vi "Localize CSM VIs.vi"(5 "API Dir":path[](array[path]), 6 "options":cluster{"Force?(F)":bool, "Show FP":bool}={"Force?(F)"=FALSE, "Show FP"=TRUE}, 7 "doc dir":path[](array[path]), 8 "error in (no error)":errorcluster, 10 "Language Ring":string(combo)="English(en-us)") -> (0 "error out":errorcluster)   [LabVIEW 2017, in "csmdoc.lvlib"]
uses:
  csmdoc.lvlib
  BEditor-Localization.vi
  _Typedef/DocElement.ctl
  _Shared/CSM Shared.lvlib
  _tool/_batchEditorDialog/batchEditorDialog.lvlib
  Communicable State Machine.lvlib
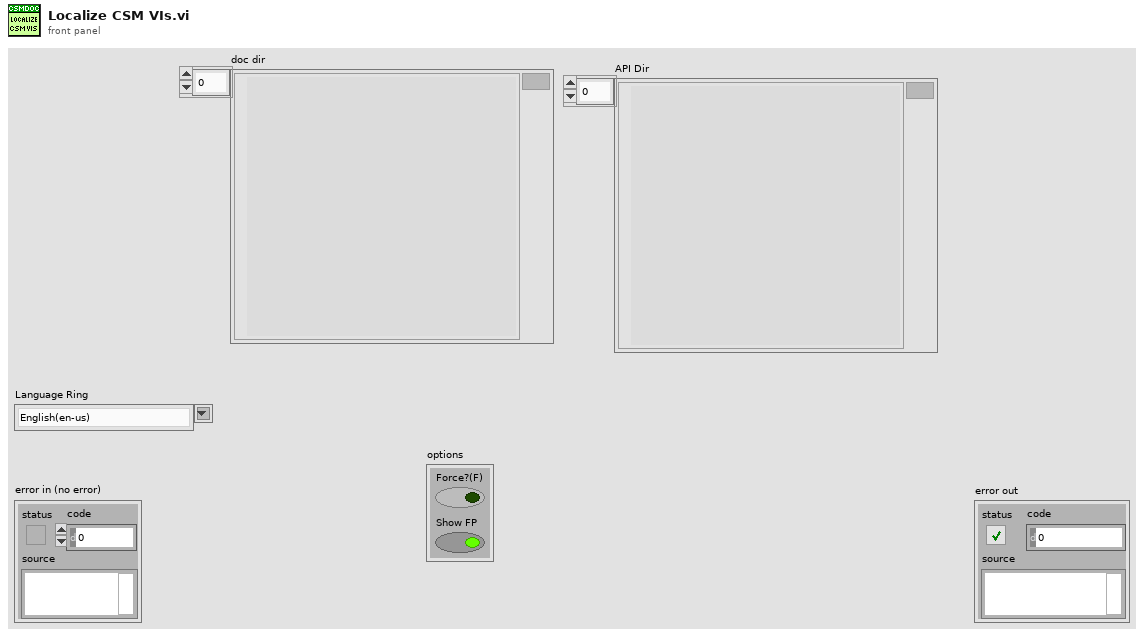
[diagram p1: front panel]
types:
  T1 = typedef "csmdoc.lvlib/DocNote.ctl" = cluster{"ID":string, "Content":string, "Type":string}
  T2 = typedef "csmdoc.lvlib/DocElement.ctl" = cluster{"ID":string, "Content":string[], "SubIDs":string[], "Path":string[]}
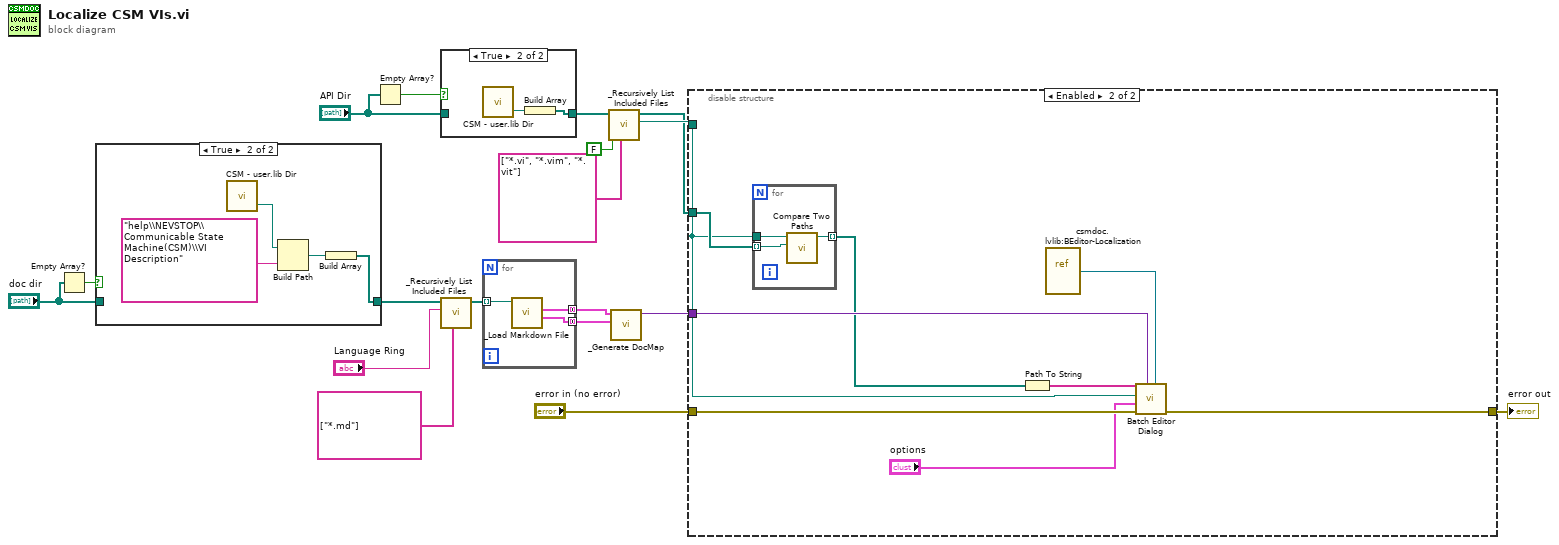
[diagram p0: block diagram]
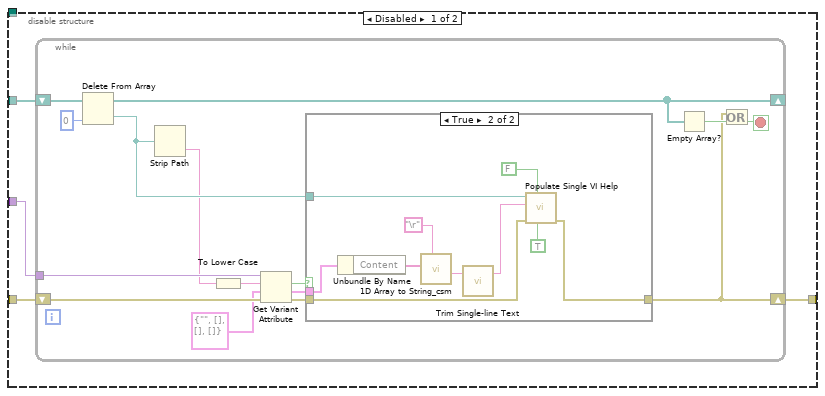
[diagram p2: hidden frame]
diagram:
  n1 = Empty Array?(array="doc dir") -> (empty?=w12:bool)
  n2 = case shown="True" w12 {
    tunnel: [w19 w20] -> w18
    tunnel: "doc dir" -> [w19 _]
    frame False {
    }
    frame True {
      n3 = call "CSM - user.lib Dir.vi"() -> ("<LabVIEW>"=w21:path)  [unwired: 2 in, 1 out]
      n4 = Build Path(base path=w21, name or relative path="help\\NEVSTOP\\Communicable State Machine(CSM)\\VI Description") -> (appended path=w22:path)
      n5 = Build Array(w22) -> (w20:path[])
    }
  }
  n6 = Empty Array?(array="API Dir") -> (empty?=w10:bool)
  n7 = case shown="True" w10 {
    tunnel: "API Dir" -> [w24 _]
    tunnel: [w24 w25] -> w3
    frame False {
    }
    frame True {
      n8 = call "CSM - user.lib Dir.vi"() -> ("<LabVIEW>"=w26:path)  [unwired: 2 in, 1 out]
      n9 = Build Array(w26) -> (w25:path[])
    }
  }
  n10 = call "_Recursively List Included Files.vi"("pattern"=string[] ["*.md"], "Language Ring"="Language Ring", "dir"=w18) -> ("Array"=w15:path[])  [unwired: 7 in, 1 out]
  n11 = for {
    tunnel: w15 -> [w29] mode=indexing
    tunnel: [w28] -> w17 mode=concatenating
    tunnel: [w27] -> w16 mode=concatenating
    n12 = call "_Load Markdown File.vi"("Path"=w29) -> ("Array 2"=w27:T1[], "Array"=w28:T2[])  [unwired: 8 in, 1 out]
  }
  n13 = call "_Recursively List Included Files.vi"("pattern"=string[] ["*.vi", "*.vim", "*.vit"], "apply _ filter?(T)"=FALSE, "dir"=w3) -> ("Common Path"=w6:path, "Array"=w4:path[])  [unwired: 7 in]
  n14 = call "_Generate DocMap.vi"("Array 2"=w16, "Array"=w17) -> ("Variant"=w13:variant)  [unwired: 9 in]
  n15 = disable-structure shown="Enabled" {
    disable-tunnel: [w33 w67] -> w14
    disable-tunnel: "error in (no error)" -> [w32 w68]
    disable-tunnel: w13 -> [w31 w66]
    disable-tunnel: w4 -> [w30 w62]
    disable-tunnel: w6 -> [_ w60]
    frame Disabled {
      n16 = while {
        shift-right: [w45] -> _
        shift-left: w30 -> [w47]
        tunnel: w31 -> [w43]
        shift-right: [w34] -> w33
        shift-left: w32 -> [w40]
        stop <- w35 stop-if-true
        n17 = Delete From Array(array=w47, index=0) -> (deleted portion=w48:path, array with subset deleted=w45:path[])  [unwired: 1 in]
        n18 = Strip Path(path=w48) -> (name=w42:string)  [unwired: 1 out]
        n19 = To Lower Case(string=w42) -> (all lower case string=w37:string)
        n20 = Get Variant Attribute(Variant=w43, name=w37, default value (empty Variant)=T2 {"ID"="", "Content"=[], "SubIDs"=[], "Path"=[]} ("Cluster"), error in=w40) -> (found=w41:bool, value=w38:T2, error out=w39:errorcluster)  [unwired: 1 out]
        n21 = case shown="True" w41 {
          tunnel: w48 -> [_ w59]
          tunnel: w39 -> [w49 w58]
          tunnel: [w49 w57] -> w34
          tunnel: w38 -> [_ w53]
          frame False {
          }
          frame True {
            n22 = Unbundle By Name(w53) -> ("Content"=w56:string[])
            n23 = call "1D Array to String_csm.vi"("delimiter (Tab)"="\r", "Array of Strings"=w56) -> ("delimited string"=w54:string)  [unwired: 9 in]
            n24 = call "Trim Single-line Text.vi"("single-line text"=w54) -> ("trimed text"=w52:string)  [unwired: 2 in]
            n25 = call "Populate Single VI Help.vi"("Show FP"=TRUE, "Force?(F)"=FALSE, "error in (no error)"=w58, "VI Description"=w52, "Path"=w59) -> ("error out"=w57:errorcluster)  [unwired: 6 in]
          }
        }
        n26 = Empty Array?(array=w45) -> (empty?=w46:bool)
        n27 = Or(x=w34, y=w46) -> (x .or. y?=w35:bool)
      }
    }
    frame Enabled {
      n28 = for {
        tunnel: w60 -> [w71]
        tunnel: w62 -> [w70] mode=indexing
        tunnel: [w69] -> w61 mode=indexing
        n29 = call <vilib>:"Compare Two Paths.vi"("Path 2"=w70, "Path 1"=w71) -> ("Relative Path from 1 to 2"=w69:path)  [unwired: 6 in, 3 out]
      }
      n30 = Path To String(path=w61) -> (string=w65:string[])
      n31 = vi-ref "csmdoc.lvlib:BEditor-Localization.vi"() -> (w64:refnum<vi>)
      n32 = call "Batch Editor Dialog.vi"("VI Refnum"=w64, "Reference"=w66, "Error in"=w68, "Option"="options", "Root"=w60, "Entries"=w65) -> ("Error out"=w67:errorcluster)  [unwired: 5 in]
    }
  }
  "error out" <- w14
